vi "Lab_view_Lab_view.vi"() -> ()   [LabVIEW 2013]
uses:
  <vilib>/Instr/_visa.llb/VISA Configure Serial Port (Instr).vi
panel:
  in  "stop":bool
  out "error out 2":errorcluster
  in  "data bits (8) 2":u16=8 min=5 max=8 step=1
  in  "baud rate (9600) 2":u32=9600
  in  "VISA resource name 2":refnum<visa-resource-name>
  out "read buffer 2":string
  in  "MODE":bool
  out "pos and status":bool
  out "position":bool
  out "control":bool
  in  "pos and status":bool
  in  "position":bool
  in  "Control":bool
  out "error out":errorcluster
  out "read buffer":string
  in  "write buffer":string
  in  "data bits (8)":u16=8 min=5 max=8 step=1
  in  "baud rate (9600)":u32=9600
  in  "VISA resource name":refnum<visa-resource-name>
  # "Text Mode"
  # "Select : ON : Text Mode , \n              OFF : ButtonMode"
  # "Button Mode"
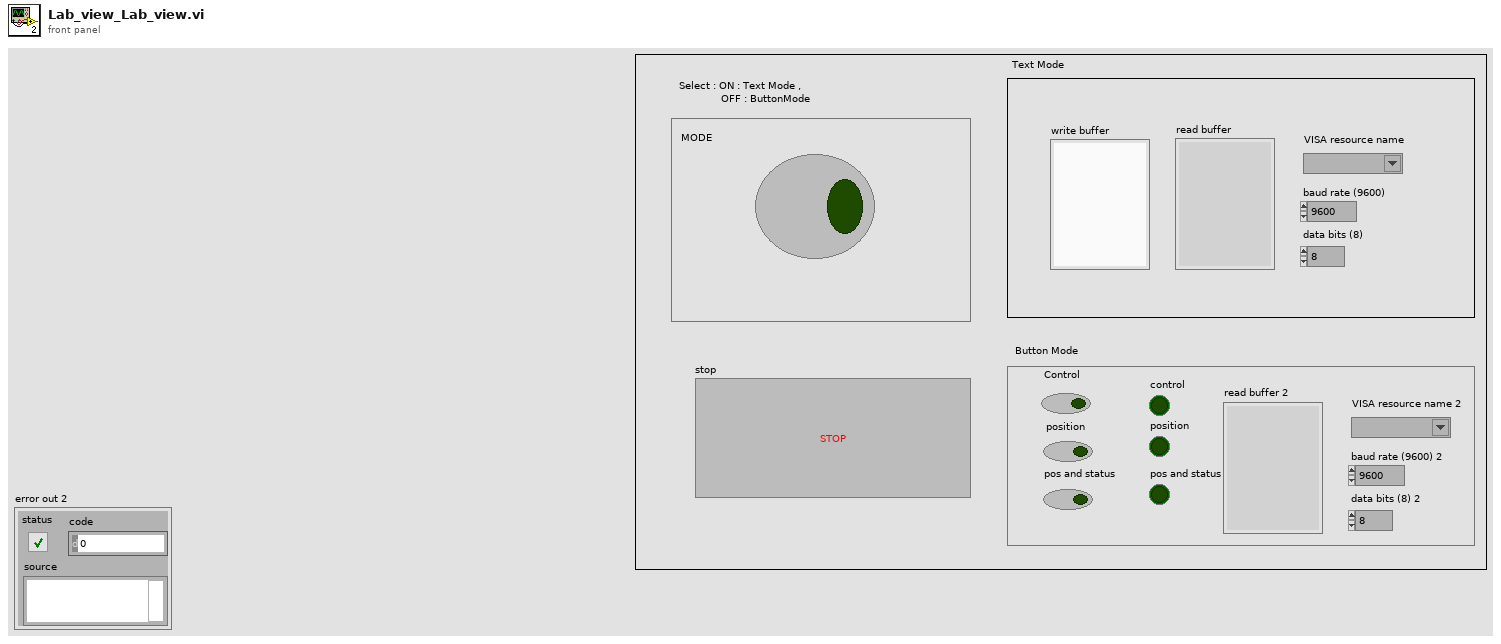
[diagram p1: front panel]
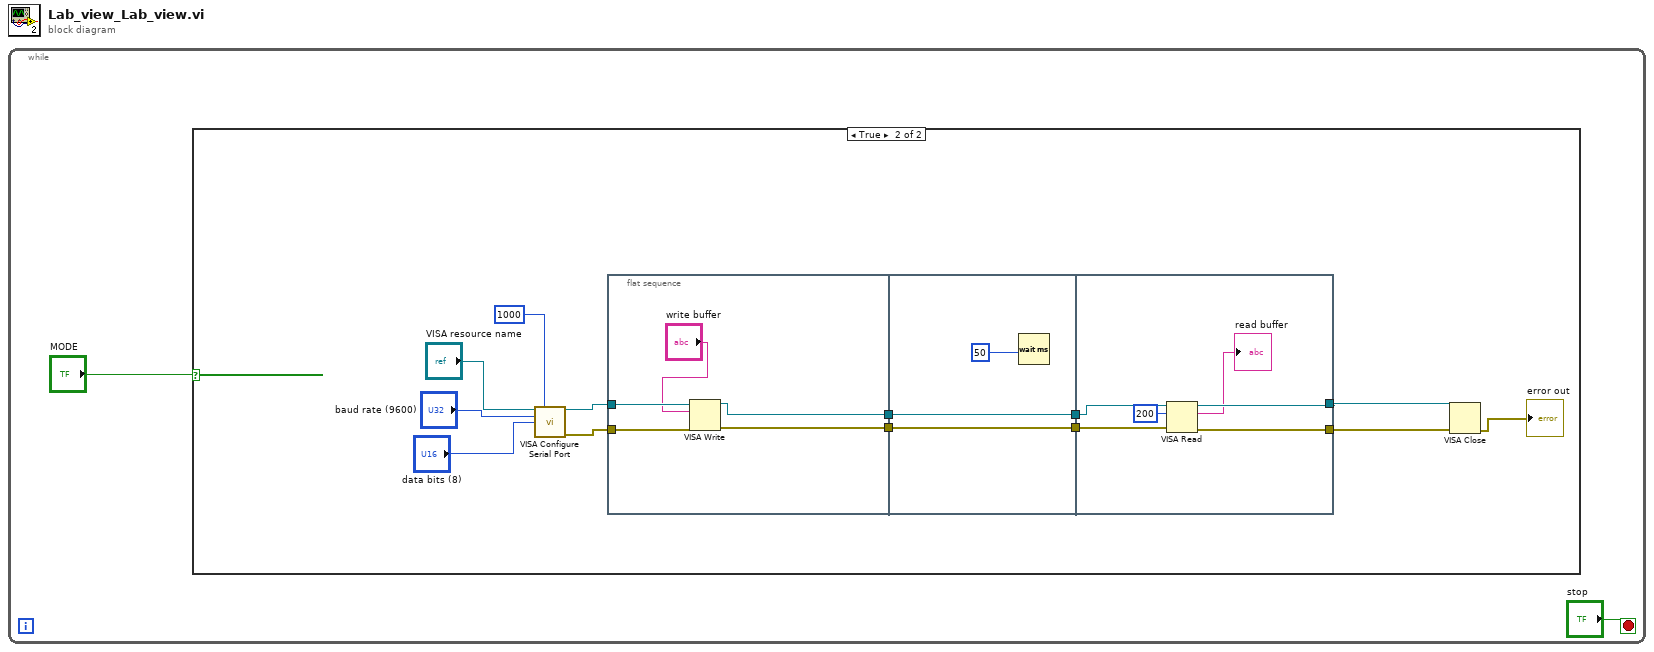
[diagram p0: block diagram]
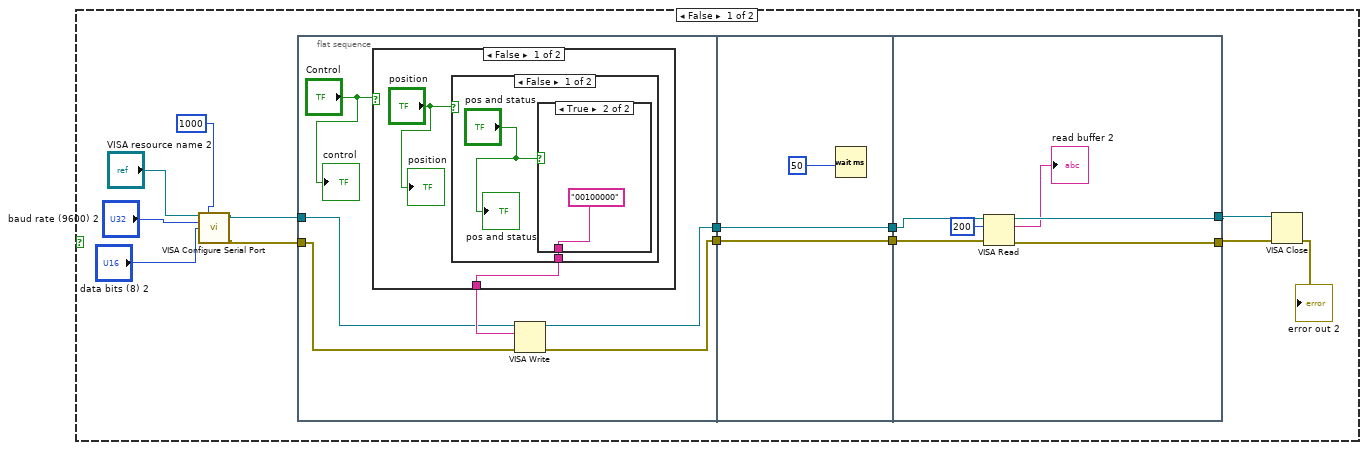
[diagram p2: hidden frame]
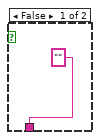
[diagram p3: hidden frame]
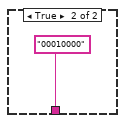
[diagram p4: hidden frame]
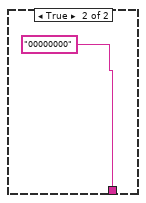
[diagram p5: hidden frame]
diagram:
  n1 = while {
    stop <- "stop" stop-if-true
    n2 = case shown="True" "MODE" {
      frame False {
        n3 = call-poly "VISA Configure Serial Port"("VISA resource name"="VISA resource name 2", "timeout (10sec)"=u32 1000, "baud rate (9600)"="baud rate (9600) 2", "data bits (8)"="data bits (8) 2") -> ("VISA resource name out"=w8:refnum<visa-resource-name>, "error out"=w7:errorcluster)  [unwired: 10 in]
        n4 = flat-sequence {
          tunnel: [w17] -> w15
          tunnel: w8 -> [w20]
          tunnel: w7 -> [w19]
          tunnel: [w18] -> w6
          tunnel: [w30] -> w14
          tunnel: [w31] -> w13
          tunnel: w15 -> [w31]
          tunnel: w6 -> [w30]
          tunnel: w14 -> [w38]
          tunnel: w13 -> [w37]
          tunnel: [w36] -> w3
          tunnel: [w35] -> w4
          frame #0 {
            n5 = case shown="False" "Control" {
              tunnel: [w23 "00000000"] -> w21
              frame False {
                n6 = case shown="False" "position" {
                  tunnel: [w25 "00010000"] -> w23
                  frame False {
                    n7 = case shown="True" "pos and status" {
                      tunnel: ["" "00100000"] -> w25
                      frame False {
                      }
                      frame True {
                      }
                    }
                    "pos and status" <- "pos and status"
                  }
                  frame True {
                  }
                }
                "position" <- "position"
              }
              frame True {
              }
            }
            n8 = VISA Write(VISA resource name=w20, write buffer=w21, error in (no error)=w19) -> (VISA resource name out=w18:refnum<visa-resource-name>, error out=w17:errorcluster)  [unwired: 1 out]
            "control" <- "Control"
          }
          frame #1 {
            n9 = Wait (ms)(milliseconds to wait=u32 50) -> ()  [unwired: 1 out]
          }
          frame #2 {
            n10 = VISA Read(VISA resource name=w38, byte count=u32 200, error in (no error)=w37) -> (VISA resource name out=w35:refnum<visa-resource-name>, read buffer=→"read buffer 2":string, error out=w36:errorcluster)  [unwired: 1 out]
          }
        }
        n11 = VISA Close(VISA resource name=w4, error in (no error)=w3) -> (error out=→"error out 2":errorcluster)
      }
      frame True {
        n12 = call-poly "VISA Configure Serial Port"("VISA resource name"="VISA resource name", "timeout (10sec)"=u32 1000, "baud rate (9600)"="baud rate (9600)", "data bits (8)"="data bits (8)") -> ("VISA resource name out"=w43:refnum<visa-resource-name>, "error out"=w42:errorcluster)  [unwired: 10 in]
        n13 = flat-sequence {
          tunnel: w43 -> [w54]
          tunnel: w42 -> [w56]
          tunnel: [w53] -> w51
          tunnel: [w55] -> w50
          tunnel: [w58] -> w49
          tunnel: w51 -> [w58]
          tunnel: [w57] -> w48
          tunnel: w50 -> [w57]
          tunnel: w49 -> [w65]
          tunnel: w48 -> [w64]
          tunnel: [w63] -> w40
          tunnel: [w62] -> w41
          frame #0 {
            n14 = VISA Write(VISA resource name=w54, write buffer="write buffer", error in (no error)=w56) -> (VISA resource name out=w53:refnum<visa-resource-name>, error out=w55:errorcluster)  [unwired: 1 out]
          }
          frame #1 {
            n15 = Wait (ms)(milliseconds to wait=u32 50) -> ()  [unwired: 1 out]
          }
          frame #2 {
            n16 = VISA Read(VISA resource name=w65, byte count=u32 200, error in (no error)=w64) -> (VISA resource name out=w62:refnum<visa-resource-name>, read buffer=→"read buffer":string, error out=w63:errorcluster)  [unwired: 1 out]
          }
        }
        n17 = VISA Close(VISA resource name=w41, error in (no error)=w40) -> (error out=→"error out":errorcluster)
      }
    }
  }
